vi "Workspace Pull UI Objects.vi"(8 "error in (no error)":errorcluster, 11 "UI.Refs":T1) -> (0 "error out":errorcluster, 2 "Values":dbl[](array[numeric]))   [LabVIEW 2015, in "Diagnostics Addon Shared.lvlib"]
uses:
  Diagnostics Addon Shared.lvlib
  Types/UI.Refs.ctl
  Types/Command.ctl
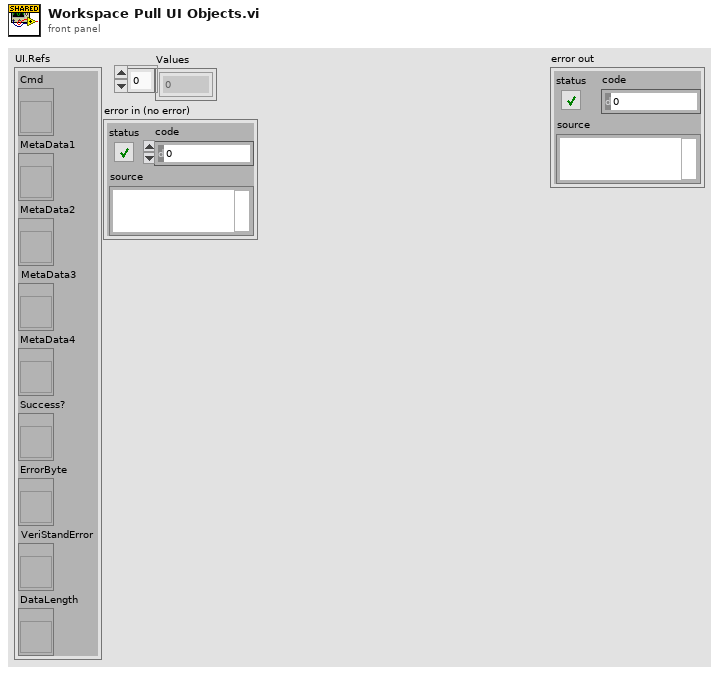
[diagram p1: front panel]
types:
  T1 = typedef "Diagnostics Addon Shared.lvlib/UI.Refs.ctl" = cluster{"Cmd":refnum<vi>, "MetaData1":refnum<vi>, "MetaData2":refnum<vi>, "MetaData3":refnum<vi>, "MetaData4":refnum<vi>, "Success?":refnum<vi>, "ErrorByte":refnum<vi>, "VeriStandError":refnum<vi>, "DataLength":refnum<vi>}
  T2 = typedef "Diagnostics Addon Shared.lvlib/Channel Commands Enum.ctl" = enum8{"None", "EnableDiagnosticSession", "DisableDiagnosticSession", "ReadDataIdentifiers", "ReadDataIdentifier", "WriteDataIndentifier", "ReadPIDsOnDemand", "ReadPIDOnDemand", "WriteCPID", "WriteMemory", "ReadMemory", "ReadDTCs", "ClearDTCs", "ControlDTC", "ForceTesterPresent", "DisableNormalCommunication", "ReturnToNormalMode", "InputOutputControl", "StartRoutine", "RequestRoutineStatus", "StopRoutine", "ECUReset", "UnlockECU", "ClearSuccessBit", "ConfigureandStartPIDs", "StopPIDs", "StartDTCs", "EnableChangeDTCCount", "DisableChangeDTCCount", "ReadFailureRecordParameters", "PassThru Channel Based"}
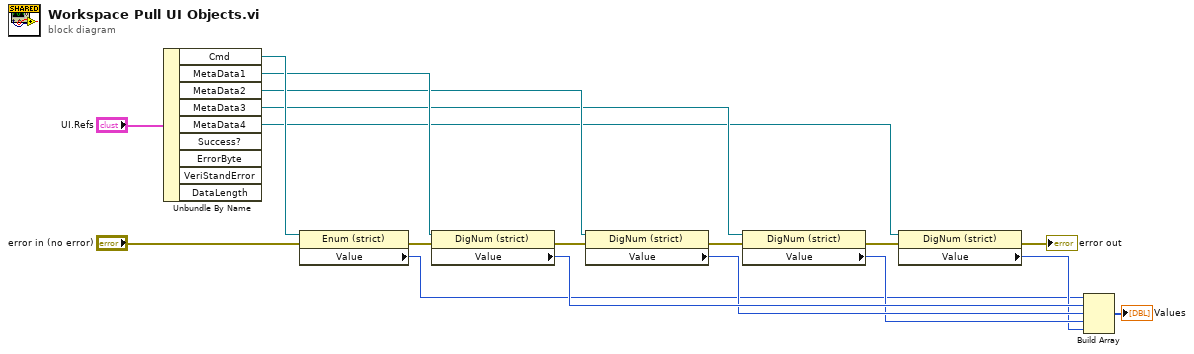
[diagram p0: block diagram]
diagram:
  n1 = Unbundle By Name("UI.Refs") -> ("Cmd"=w17:refnum<vi>, "MetaData1"=w16:refnum<vi>, "MetaData2"=w15:refnum<vi>, "MetaData3"=w14:refnum<vi>, "MetaData4"=w10:refnum<vi>)  [unwired: 4 out]
  n2 = property class="Enum (strict)"(reference=w17, error in="error in (no error)") -> (error out=w13:errorcluster, "Value"=w1:T2)  [unwired: 1 out]
  n3 = property class="DigNum (strict)"(reference=w16, error in=w13) -> (error out=w12:errorcluster, "Value"=w6:i64)  [unwired: 1 out]
  n4 = property class="DigNum (strict)"(reference=w15, error in=w12) -> (error out=w11:errorcluster, "Value"=w5:i64)  [unwired: 1 out]
  n5 = property class="DigNum (strict)"(reference=w14, error in=w11) -> (error out=w9:errorcluster, "Value"=w4:i64)  [unwired: 1 out]
  n6 = property class="DigNum (strict)"(reference=w10, error in=w9) -> (error out=→"error out":errorcluster, "Value"=w3:i64)  [unwired: 1 out]
  n7 = Build Array(w1, w6, w5, w4, w3) -> (→"Values":i64[])
